vi "Write Column Headers.vi"(10 "Column Headers":string[](array[string]), 11 "Logger in":refnum<class "Log.lvclass">) -> (3 "Logger out":refnum<class "Log.lvclass">)   [LabVIEW 2013, in "Log.lvclass"]
uses:
  Log.lvclass
  Log.lvclass/Log.ctl
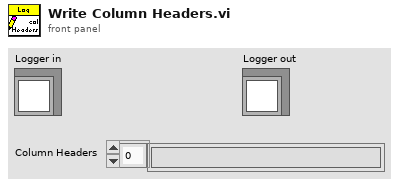
[diagram p1: front panel]
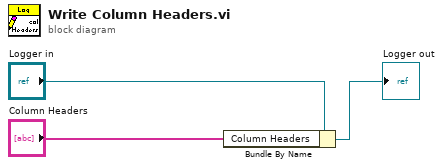
[diagram p0: block diagram]
diagram:
  n1 = Bundle By Name(cluster="Logger in", "Column Headers"="Column Headers") -> (→"Logger out":refnum<class "Log.lvclass">)
